vi "Remove BC.vi"(8 "error in":errorcluster, 11 "Target in":refnum<k24>) -> (0 "error out":errorcluster, 3 "Target out":refnum<k24>)   [LabVIEW 2020]
uses:
  NationalInstruments.VeriStand.SystemDefinitionAPI
  Scripting/AIM MIL-STD-1553 Scripting.lvlib
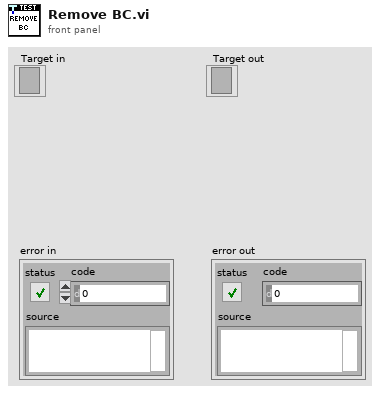
[diagram p1: front panel]
types:
  T1 = typedef "Custom Device API.lvlib/Custom Device Item Ref.ctl" = u64
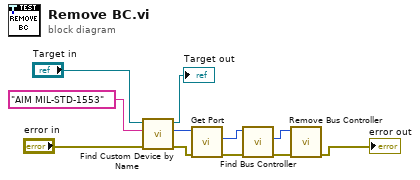
[diagram p0: block diagram]
diagram:
  n1 = call "Find Custom Device by Name.vi"("error in"="error in", "custom device name"="AIM MIL-STD-1553" ("name"), "target"="Target in") -> ("error out"=w10:errorcluster, "custom device"=w11:T1, "target out"=→"Target out":refnum<k24>)  [unwired: 5 in, 1 out]
  n2 = call "Get Port.vi"("error in"=w10, "custom device ref"=w11) -> ("error out"=w9:errorcluster, "port"=w8:T1)  [unwired: 6 in, 2 out]
  n3 = call "Find Bus Controller.vi"("error in"=w9, "port"=w8) -> ("error out"=w6:errorcluster, "bus controller"=w7:T1)  [unwired: 6 in, 2 out]
  n4 = call "Remove Bus Controller.vi"("error in"=w6, "bus controller"=w7) -> ("error out"=→"error out":errorcluster)  [unwired: 9 in]
